vi "mod_SSB filter design.vi"(0 "hilbert filter":T1={"taps"=81, "design"=enum."Windowed Hilbert Transformer"}, 5 "side-band":enum16{"Lower sideband", "Upper sideband"}(ring), 11 "error in (no error)":errorcluster, 13 "reset? (T)":bool=TRUE) -> (4 "AM-SSB filter taps":cdb[](array[numeric]), 15 "error out":errorcluster)   [LabVIEW 2020, in "niAMT.lvlib"]
uses:
  <vilib>/addons/Modulation/niAMT.lvlib
  <vilib>/addons/Modulation/Analog/controls/mod_Hilbert filter.ctl
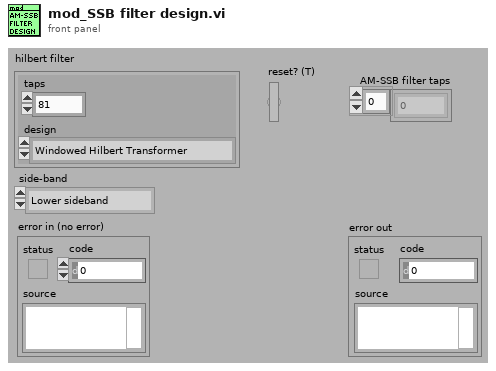
[diagram p1: front panel]
types:
  T1 = typedef "niAMT.lvlib/mod_Hilbert filter.ctl" = cluster{"taps":i32, "design":enum16{"Windowed Hilbert Transformer", "Equiripple Hilbert transformer"}}
  T2 = enum16{"Windowed Hilbert Transformer", "Equiripple Hilbert transformer"}
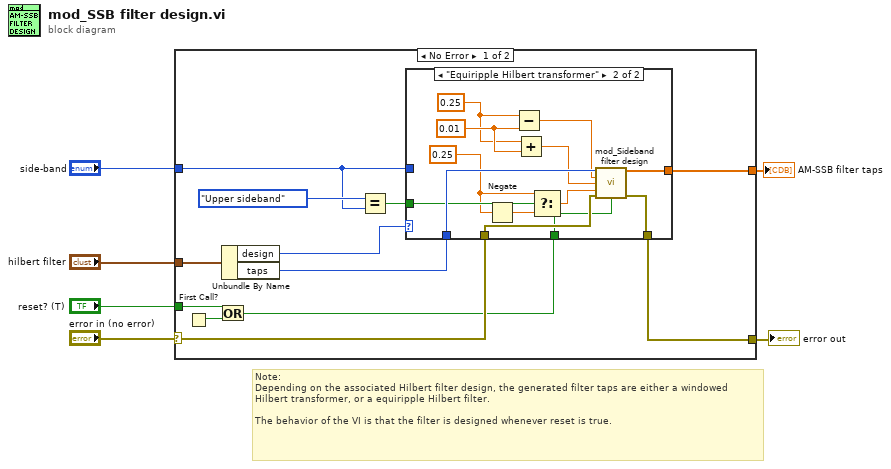
[diagram p0: block diagram]
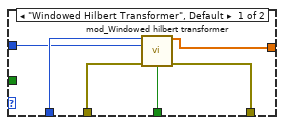
[diagram p2: hidden frame]
diagram:
  # "Note:\nDepending on the associated Hilbert filter design, the generated filter taps are either a windowed\nHilbert transformer, or a equiripple Hilbert filter.\n\nThe behavior of the VI is that the filter is designed whenever reset is true."
  n1 = case shown="No Error" "error in (no error)" {
    selector: "error in (no error)" -> [w16 w38]
    tunnel: "hilbert filter" -> [w18 _]
    tunnel: "side-band" -> [w8 _]
    tunnel: "reset? (T)" -> [w13 _]
    tunnel: [w11 _] -> w2
    tunnel: [w10 w38] -> w1
    frame No Error {
      n2 = First Call?() -> (First Call?: T/F=w14:bool)
      n3 = Or(x=w13, y=w14) -> (x .or. y?=w12:bool)
      n4 = Unbundle By Name(w18) -> ("design"=w15:T2, "taps"=w17:i32)
      n5 = Equal?(x=enum16{"Lower sideband", "Upper sideband"}."Upper sideband" ("Side-band"), y=w8) -> (x = y?=w7:bool)
      n6 = case shown="\"Equiripple Hilbert transformer\"" w15 {
        tunnel: [w24 w37] -> w10
        tunnel: [w23 w35] -> w11
        tunnel: w17 -> [w22 w34]
        tunnel: w8 -> [w21 _]
        tunnel: w16 -> [w20 w32]
        tunnel: w12 -> [w19 w31]
        tunnel: w7 -> [_ w33]
        frame "Windowed Hilbert Transformer", Default {
          n7 = call <vilib>:"mod_Windowed hilbert transformer.vi"("filter taps"=w22, "side-band"=w21, "error in (no error)"=w20, "reset? (T)"=w19) -> ("hilbert transformer taps"=w23:cdb[], "error out"=w24:errorcluster)  [unwired: 10 out]
        }
        frame "Equiripple Hilbert transformer" {
          w26 = 0.25
          w27 = 0.01
          w25 = 0.25
          n8 = Negate(x=w26) -> (-x=w36:dbl)
          n9 = Subtract(x=w25, y=w27) -> (x-y=w29:dbl)
          n10 = Add(x=w25, y=w27) -> (x+y=w28:dbl)
          n11 = Select(t=w26, s=w33, f=w36) -> (s? t:f=w30:dbl)
          n12 = call <vilib>:"mod_Sideband filter design.vi"("taps"=w34, "lower pass band frequency"=w29, "lower stop band frequency"=w28, "frequency shift"=w30, "error in (no error)"=w32, "reset? (T)"=w31) -> ("filter taps"=w35:cdb[], "error out"=w37:errorcluster)  [unwired: 8 out]
        }
      }
    }
    frame Error {
    }
  }
  "AM-SSB filter taps" <- w2
  "error out" <- w1
